vi "MidiWrapperPlayground.vi"() -> ()   [LabVIEW 2020]
uses:
  x64/Release/MIDIInToLabVIEWWrapper.dll
panel:
  out "phMidiIn":u64
  out "Data2":i32
  out "Data1":i32
  out "Status":i32
  out "error out":errorcluster
  out "error 4":i32
  out "error 3":i32
  out "error 2":i32
  out "error":i32
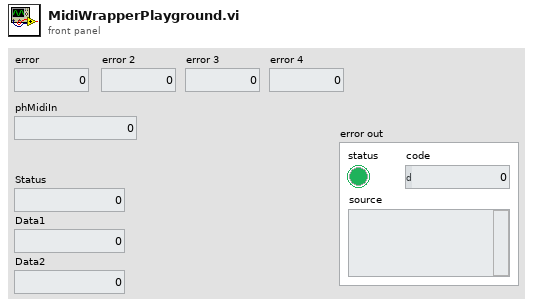
[diagram p1: front panel]
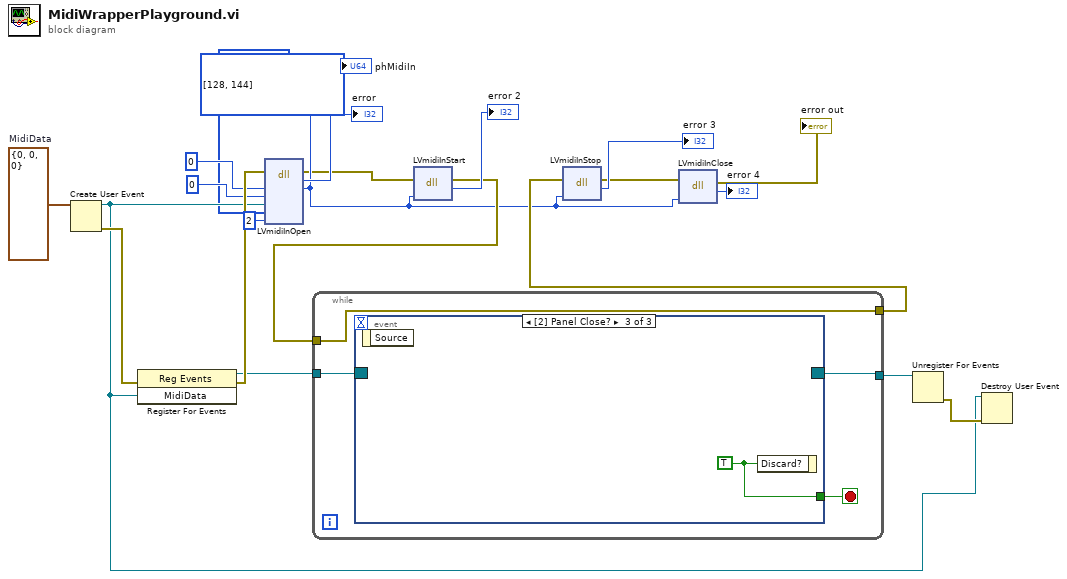
[diagram p0: block diagram]
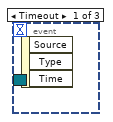
[diagram p2: hidden frame]
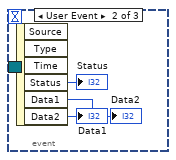
[diagram p3: hidden frame]
diagram:
  w5 = cluster{"Status":i32, "Data1":i32, "Data2":i32} {"Status"=0, "Data1"=0, "Data2"=0}  # MidiData
  n1 = Create User Event(user event datatype=w5) -> (user event=w8:refnum<user-event>, error out=w13:errorcluster)  [unwired: 1 in]
  n2 = register-events(error in=w13, w8) -> (reference out=w11:refnum<event-registration>, error out=w12:errorcluster)  [unwired: 1 in]
  n3 = dll-call lib="C:/code/LabVIEW-MIDI/cpp-src/MIDIInToLabVIEWWrapper/x64/Release/MIDIInToLabVIEWWrapper.dll" fn="LVmidiInOpen"(error in=w12, "phMidiIn"=u64 0 ("hMidiIn"), "uDeviceID"=u32 0, "pUserEventRef"=w8, "filterArray"=u8[] [128, 144], "arraySize"=2) -> (error out=w1:errorcluster, "error"=→"error":i32, "phMidiIn"=w4:u64)  [unwired: 6 in, 1 out]
  "phMidiIn" <- w4
  n4 = dll-call lib="C:/code/LabVIEW-MIDI/cpp-src/MIDIInToLabVIEWWrapper/x64/Release/MIDIInToLabVIEWWrapper.dll" fn="LVmidiInStart"(error in=w1, "hMidiIn"=w4) -> (error out=w15:errorcluster, "error"=→"error 2":i32)  [unwired: 3 in, 1 out]
  n5 = while {
    tunnel: w15 -> [w24]
    tunnel: [w24] -> w14
    tunnel: w11 -> [w23]
    tunnel: [w22] -> w10
    stop <- w25 stop-if-true
    n6 = event shown="[2] Panel Close?" {
      selector: w23 -> [_ _ _]
      dyn-events: [_ _ _] -> w22
      timeout: _ -> [_ _ _]
      tunnel: [_ _ w29] -> w25
      event Timeout {
        n7 = event-data() -> ()  [unwired: 1 in, 3 out]
      }
      event User Event {
        n8 = event-data() -> ("Status"=→"Status":i32, "Data1"=→"Data1":i32, "Data2"=→"Data2":i32)  [unwired: 1 in, 3 out]
      }
      event Panel Close? {
        w29 = TRUE ("Discard?")
        n9 = event-data() -> ()  [unwired: 1 in, 1 out]
        n10 = event-data("Discard?"=w29) -> ()  [unwired: 1 in, 1 out]
      }
    }
  }
  n11 = dll-call lib="C:/code/LabVIEW-MIDI/cpp-src/MIDIInToLabVIEWWrapper/x64/Release/MIDIInToLabVIEWWrapper.dll" fn="LVmidiInStop"(error in=w14, "hMidiIn"=w4) -> (error out=w17:errorcluster, "error"=→"error 3":i32)  [unwired: 3 in, 1 out]
  n12 = dll-call lib="C:/code/LabVIEW-MIDI/cpp-src/MIDIInToLabVIEWWrapper/x64/Release/MIDIInToLabVIEWWrapper.dll" fn="LVmidiInClose"(error in=w17, "hMidiIn"=w4) -> (error out=→"error out":errorcluster, "error"=→"error 4":i32)  [unwired: 3 in, 1 out]
  n13 = Unregister For Events(event registration refnum=w10) -> (error out=w9:errorcluster)  [unwired: 1 in]
  n14 = Destroy User Event(user event=w8, error in=w9) -> ()  [unwired: 1 out]
